vi "Count down.vi"(8 "error in (no error)":errorcluster caption="错误输入（无错误）", 11 "Time":i32) -> (0 "error out":errorcluster caption="错误输出")   [LabVIEW 2018]
panel:
  out "Move will start in...":i32
  # "秒后Z轴开始向下运动"
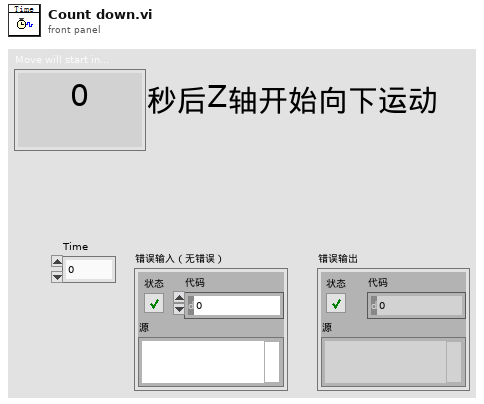
[diagram p1: front panel]
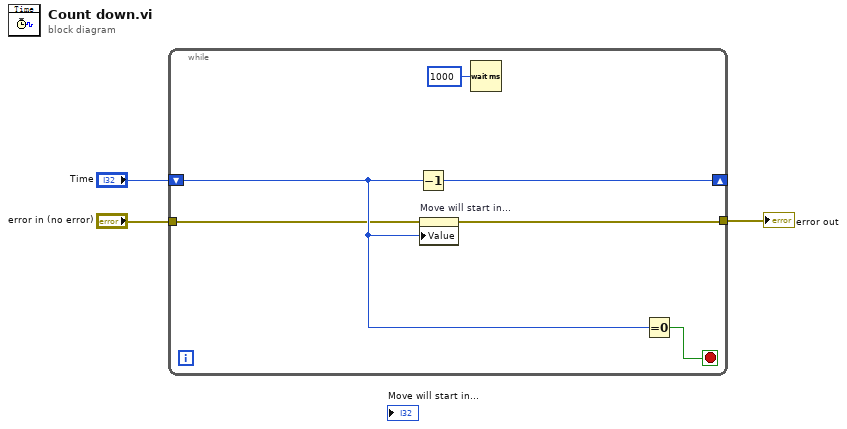
[diagram p0: block diagram]
diagram:
  n1 = while {
    shift-right: [w9] -> _
    shift-left: "Time" -> [w7]
    tunnel: "error in (no error)" -> [w5]
    tunnel: [w4] -> w1
    stop <- w6 stop-if-true
    n2 = Decrement(x=w7) -> (x-1=w9:i32)
    n3 = property on="Move will start in..." class="DigNum (严格)"(error in=w5, "Value"=w7) -> (error out=w4:errorcluster)  [unwired: 1 in, 1 out]
    n4 = Wait (ms)(milliseconds to wait=u32 1000 ("等待时间（毫秒）")) -> ()  [unwired: 1 out]
    n5 = Equal To 0?(x=w7) -> (x = 0?=w6:bool)
  }
  "error out" <- w1
